vi "振动检测.vi"(0 "振动一":refnum<vi>, 1 "通道输入":tag="cDAQ2Mod1/ai0", 5 "振动二":refnum<vi>, 7 "重置":bool, 11 "error in":errorcluster caption="错误输入") -> (4 "spectrum info":T1[](array[typedef]) {"x-axis units" items=["Time (s)"=0, "Frequency-CB (Hz)"=1, "Frequency-CPB (Hz)"=1248, "Frequency-Arbitrary (Hz)"=2357, "Quefrency (s)"=2, "Revolutions (rev)"=3, "Order"=4, "Speed (RPM)"=11, "Speed (rad/s)"=21, "Index"=65535]; "weighting filter" items=["Linear", "A-weighting", "B-weighting", "C-weighting", "ITU-R 468-4", "Dolby", "CCITT", "C-message", "Wb", "Wc", "Wd", "We", "Wf", "Wh", "Wj", "Wk", "Wm", "AES17 20 kHz lowpass", "AES17 40 kHz lowpass", "AES17 20 kHz highpass", "AES17 40 kHz highpass"]; "dB reference [EU]" format="%.2f"; "engineering units" items=["custom..."=0, "V"=1, "A"=21, "C"=30, "pC"=31, "s"=32, "-"=29, "Pa"=2, "N"=20, "g"=3, "m/s^2"=4, "m/s"=5, "m"=6, "mm/s"=12, "mm"=13, "micron/s"=14, "micron"=15, "in/s^2"=7, "in/s"=8, "in"=9, "mil/s"=10, "mil"=11, "rad/s^2"=16, "rad/s"=17, "rad"=18, "deg/s^2"=26, "deg/s"=27, "deg"=28, "RPM"=22, "cycle/s^2"=23, "Hz"=24, "cycle"=25, "strain"=19]; "spectral info"."window" items=["None "=0, "Hanning"=1, "Hamming"=2, "Blackman-Harris"=3, "Exact Blackman"=4, "Blackman"=5, "Flat Top"=6, "4 Term B-Harris "=7, "7 Term B-Harris"=8, "Low Sidelobe"=9, "Force - Exponential"=10, "Gaussian"=62]}, 15 "error out":errorcluster caption="错误输出")   [LabVIEW 2020]
uses:
  Global_Variable/Global.vi
  <vilib>/addons/_NISVFA/_Shared subVIs/Controls/svc_Spectrum Type.ctl
  <vilib>/addons/_NISVFA/_Shared subVIs/Controls/svc_Engineering Units Text Ring.ctl
  <vilib>/addons/_NISVFA/_Shared subVIs/Controls/svc_Weighting Filter Text Ring.ctl
  <vilib>/addons/_NISVFA/_Shared subVIs/Controls/svc_X-Axis Units.ctl
  <vilib>/addons/_NISVFA/_Shared subVIs/Controls/svc_Complimentary Spectrum Units.ctl
  <vilib>/addons/_NISVFA/_Shared subVIs/Controls/svc_Spectrum Info.ctl
panel:
  in  "扫描速率[S/s]":dbl=15000.0 min=0.0 format="%.2f"
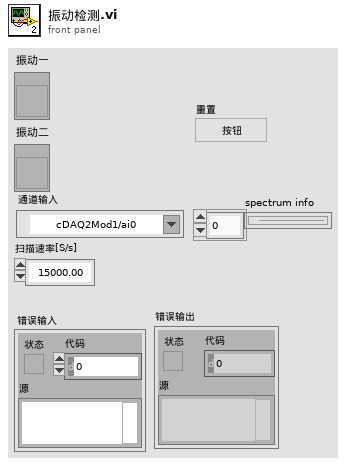
[diagram p1: front panel]
types:
  T1 = typedef "svc_Spectrum Info.ctl" = cluster{"channel name":string, "description":string, "x-axis units":T2, "spectral info":cluster{"spectrum type":T3, "linear/dB":enum16{"linear", "dB"}, "window":u16, "window size":i32, "FFT size":i32}, "engineering units":T4, "custom label":string, "dB reference [EU]":dbl, "peak units":enum16{"rms", "peak", "peak-peak"}, "weighting filter":T5, "spectral density?":bool, "unit label":string, "spectrum skewed?":bool, "complimentary spectrum units":T6}
  T2 = typedef "svc_X-Axis Units.ctl" = u16
  T3 = typedef "svc_Spectrum Type.ctl" = enum16{"FFT Spectrum [complex]", "Amplitude [Magnitude]", "Power [Magnitude^2]", "Cross Spectrum [complex]", "Frequency Response [Complex]"}
  T4 = typedef "svc_Engineering Units Text Ring.ctl" = u16
  T5 = typedef "svc_Weighting Filter Text Ring.ctl" = u16
  T6 = typedef "svc_Complimentary Spectrum Units.ctl" = enum16{"none", "radians", "degrees", "cycles", "imaginary"}
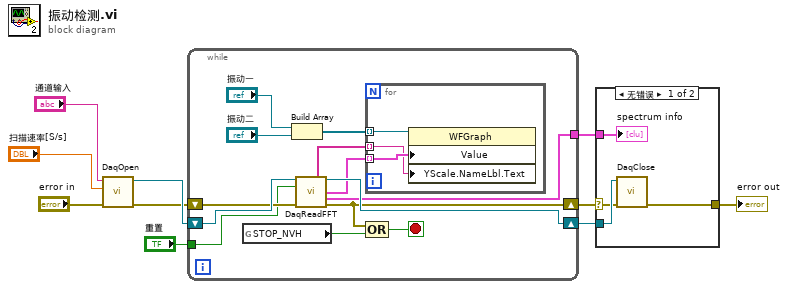
[diagram p0: block diagram]
diagram:
  n1 = call "DaqOpen.vi"("error in"="error in", "扫描速率[S/s]"="扫描速率[S/s]", "通道输入"="通道输入") -> ("error out"=w2:errorcluster, "task out"=w10:refnum<k21>)  [unwired: 7 in]
  n2 = while {
    shift-right: [w22] -> w9
    shift-left: w10 -> [w23]
    shift-right: [w21] -> w8
    shift-left: w2 -> [w18]
    tunnel: [w19] -> w5
    tunnel: "重置" -> [w12]
    stop <- w20 stop-if-true
    n3 = global read "Global.vi" "STOP_NVH"() -> (w17:bool)
    n4 = Build Array("振动一", "振动二") -> (w13:refnum<vi>[])
    n5 = call "DaqReadFFT.vi"("任务输入"=w23, "restart averaging (F)"=w12, "error in"=w18) -> ("unit labels"=w11:string[], "task out 2"=w22:refnum<k21>, "power spectra [dB EU]"=w14:cluster{"f0":dbl, "df":dbl, "magnitude":dbl[]}[], "spectrum info"=w19:T1[], "error out"=w21:errorcluster)  [unwired: 7 in, 1 out]
    n6 = for {
      tunnel: w14 -> [w25] mode=indexing
      tunnel: w13 -> [w26] mode=indexing
      tunnel: w11 -> [w24] mode=indexing
      n7 = property class="WFGraph"(reference=w26, "Value"=w25, "YScale.NameLbl.Text"=w24) -> ()  [unwired: 1 in, 2 out]
    }
    n8 = Compound Arithmetic op=OR ("复合运算")(w21, w17) -> (w20:bool)
  }
  n9 = case shown="无错误" w8 {
    selector: w8 -> [w29 w31]
    tunnel: w9 -> [w30 _]
    tunnel: [w28 w31] -> w7
    tunnel: w5 -> [w27 _]
    frame No Error {
      n10 = call "DaqClose.vi"("error in"=w29, "task in"=w30) -> ("error out"=w28:errorcluster)  [unwired: 9 in]
      "spectrum info" <- w27
    }
    frame Error {
    }
  }
  "error out" <- w7
